vi "Load and Run SubVIs for SubPanel.vi"(8 "error in (no error)":errorcluster) -> (0 "error out":errorcluster, 3 "subVIs Ref.":refnum<vi>[](array[refnum]))   [LabVIEW 2017, in "Konfiguracja.lvlib"]
doc: "Wczytuje do pamięci i uruchamia subVIs, które potem można wyświetlać w subpanelu aplikacji nadrzędnej.\nUwaga! Scieżka do subVIs to Application Directory + folder, w którym zapisane są subVIs."
uses:
  Konfiguracja.lvlib
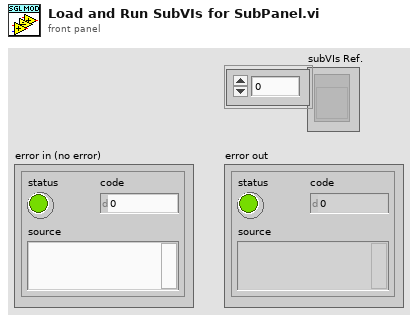
[diagram p1: front panel]
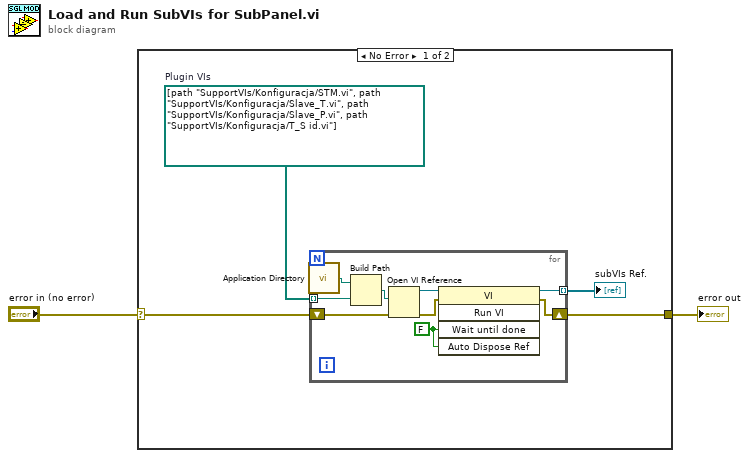
[diagram p0: block diagram]
diagram:
  n1 = case shown="No Error" "error in (no error)" {
    selector: "error in (no error)" -> [w3 w16]
    tunnel: [w6 w16] -> w2
    frame No Error {
      w4 = path[] [path "SupportVIs/Konfiguracja/STM.vi", path "SupportVIs/Konfiguracja/Slave_T.vi", path "SupportVIs/Konfiguracja/Slave_P.vi", path "SupportVIs/Konfiguracja/T_S id.vi"]  # Plugin VIs
      n2 = for {
        tunnel: w4 -> [w9] mode=indexing
        tunnel: [w13] -> w5 mode=indexing
        shift-right: [w11] -> w6
        shift-left: w3 -> [w12]
        w10 = FALSE ("Wait Until Done")
        n3 = call <vilib>:"Application Directory.vi"() -> ("Application Directory"=w7:path)
        n4 = Build Path(base path=w7, name or relative path=w9) -> (appended path=w8:path)
        n5 = Open VI Reference(vi path=w8, error in (no error)=w12) -> (vi reference=w15:refnum<vi>, error out=w14:errorcluster)  [unwired: 4 in]
        n6 = invoke class="VI" method="Run VI"(reference=w15, error in=w14, "Wait until done"=w10, "Auto Dispose Ref"=w10) -> (reference out=w13:refnum<vi>, error out=w11:errorcluster)  [unwired: 1 in, 3 out]
      }
      "subVIs Ref." <- w5
    }
    frame Error {
    }
  }
  "error out" <- w2
